vi "Stop Device.vi"(8 "error in":errorcluster, 11 "Meerstetter TEC in":refnum<class "Meerstetter TEC.lvclass">) -> (0 "error out":errorcluster, 3 "Meerstetter TEC out":refnum<class "Meerstetter TEC.lvclass">)   [LabVIEW 2014, in "Meerstetter Lib.lvlib" / "Meerstetter TEC.lvclass"]
uses:
  Meerstetter TEC.lvclass
  Meerstetter TEC.lvclass/Meerstetter TEC.ctl
  reusable/Session APIs/Serial/Serial Session.lvclass
  Configurable Device/Configurable Device.lvclass
  <userlib>/_Session Fwk/Session - Root.lvclass
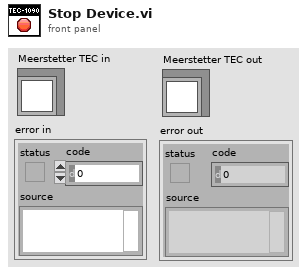
[diagram p1: front panel]
types:
  T1 = typedef "Session - Root.lvclass/Session Handle.ctl" = refnum<data-value>
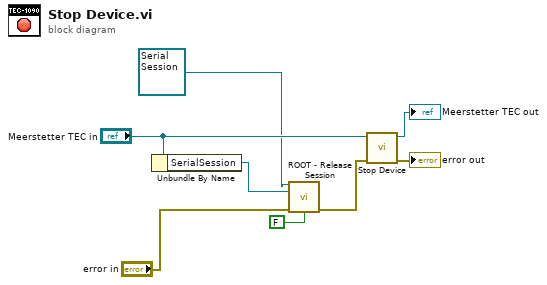
[diagram p0: block diagram]
diagram:
  n1 = Unbundle By Name("Meerstetter TEC in") -> ("SerialSession"=w5:T1)
  n2 = call <userlib>:"ROOT - Release Session.vi"("OBJ - Session in"=refnum<class "Serial Session.lvclass"> refnum ("Serial Session"), "Session Handle in"=w5, "error in (no error)"="error in", "force destroy? (F)"=FALSE) -> ("error out"=w1:errorcluster)  [unwired: 10 in, 1 out]
  n3 = call-parent "Stop Device.vi"("error in"=w1, "Configurable Device in"="Meerstetter TEC in") -> ("error out"=→"error out":errorcluster, "Configurable Device out"=→"Meerstetter TEC out":refnum<class "Meerstetter TEC.lvclass">)  [unwired: 8 in]
